vi "_PC_MS_SubVI updateTICData.vi"(7 "ydata":sgl[][](array[numeric]), 8 "error in (no error)":errorcluster, 10 "element":waveform(sgl), 11 "TIC Graph":refnum<vi>) -> (0 "error out":errorcluster)   [LabVIEW 2018]
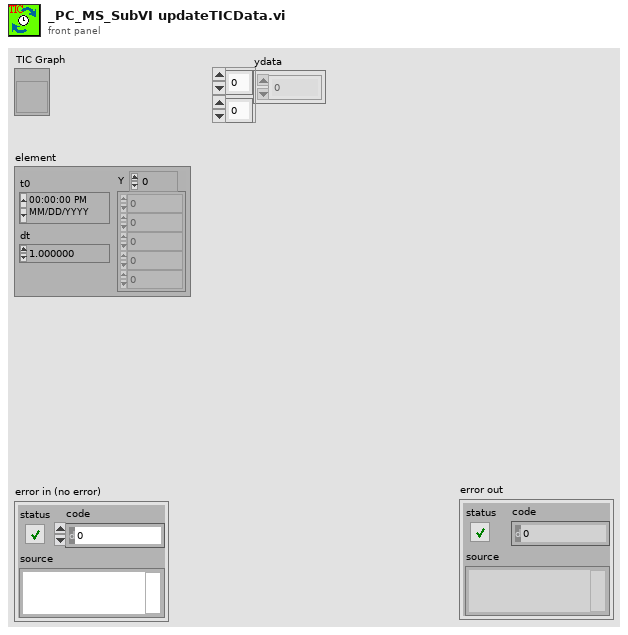
[diagram p1: front panel]
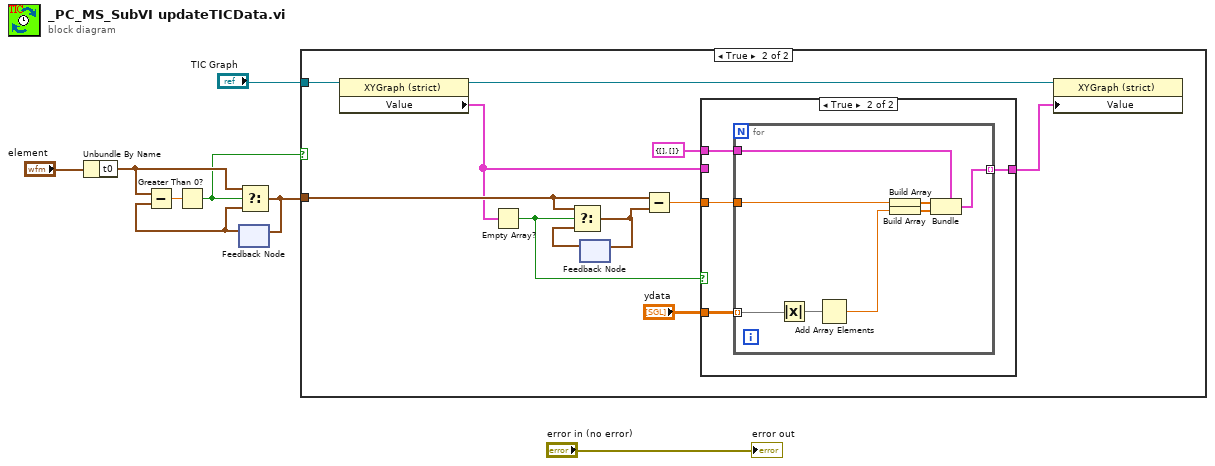
[diagram p0: block diagram]
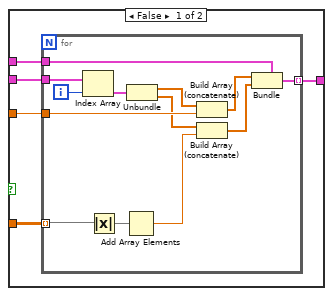
[diagram p3: hidden frame]
diagram:
  n1 = Unbundle By Name("element") -> ("t0"=w5:timestamp)
  n2 = feedback #1() -> (w6:timestamp)  [unwired: 1 in]
  n3 = Subtract(x=w5, y=w6) -> (x-y=w7:dbl)
  n4 = Greater Than 0?(x=w7) -> (x > 0?=w4:bool)
  n5 = Select(t=w5, s=w4, f=w6) -> (s? t:f=w2:timestamp)
  n6 = feedback-in #1(w2) -> ()
  n7 = case shown="True" w4 {
    tunnel: "TIC Graph" -> [_ w19]
    tunnel: w2 -> [_ w16]
    frame False {
    }
    frame True {
      n8 = property class="XYGraph (strict)"(reference=w19) -> (reference out=w12:refnum<vi>, "Value"=w14:cluster{dbl[], sgl[]}[])  [unwired: 1 in, 1 out]
      n9 = Empty Array?(array=w14) -> (empty?=w11:bool)
      n10 = feedback #2() -> (w18:timestamp)  [unwired: 1 in]
      n11 = Select(t=w16, s=w11, f=w18) -> (s? t:f=w17:timestamp)
      n12 = feedback-in #2(w17) -> ()
      n13 = Subtract(x=w16, y=w17) -> (x-y=w15:dbl)
      n14 = case shown="True" w11 {
        tunnel: "ydata" -> [w24 w40]
        tunnel: w15 -> [w23 w41]
        tunnel: w14 -> [w22 _]
        tunnel: [w21 w39] -> w13
        tunnel: cluster{dbl[], sgl[]} {[], []} -> [w20 w38]
        frame False {
          n15 = for {
            tunnel: w24 -> [w25] mode=indexing
            tunnel: w23 -> [w37]
            tunnel: w22 -> [w31]
            tunnel: [w33] -> w21 mode=indexing
            tunnel: w20 -> [w32]
            i -> [w30]
            n16 = Index Array(array=w31, index=w30) -> (element=w29:cluster{dbl[], sgl[]})
            n17 = Absolute Value(x=w25) -> (abs(x)=w26:sgl[])
            n18 = Add Array Elements(numeric array=w26) -> (sum=w36:sgl)
            n19 = Unbundle(w29) -> (w28:dbl[], w27:sgl[])
            n20 = Build Array (concatenate)(w28, w37) -> (w35:dbl[])
            n21 = Build Array (concatenate)(w27, w36) -> (w34:sgl[])
            n22 = Bundle(cluster=w32, w35, w34) -> (w33:cluster{dbl[], sgl[]})
          }
        }
        frame True {
          n23 = for {
            tunnel: w40 -> [w42] mode=indexing
            tunnel: [w49] -> w39 mode=indexing
            tunnel: w41 -> [w48]
            tunnel: w38 -> [w44]
            n24 = Absolute Value(x=w42) -> (abs(x)=w43:sgl[])
            n25 = Add Array Elements(numeric array=w43) -> (sum=w46:sgl)
            n26 = Build Array(w48) -> (w47:dbl[])
            n27 = Build Array(w46) -> (w45:sgl[])
            n28 = Bundle(cluster=w44, w47, w45) -> (w49:cluster{dbl[], sgl[]})
          }
        }
      }
      n29 = property class="XYGraph (strict)"(reference=w12, "Value"=w13) -> ()  [unwired: 1 in, 2 out]
    }
  }
  "error out" <- "error in (no error)"
